vi "get Data Read.vi"(7 "data_pos":u16, 8 "error in (no error)":errorcluster, 9 "data_length":u16, 10 "protocol_version":i32, 11 "port_num":i32) -> (0 "error out":errorcluster, 3 "function return":u32)   [LabVIEW 2022 SP3, in "dxl.lvlib"]
doc: "WINDECLSPEC uint32_t getDataRead (int port_num, int protocol_version, uint16_t data_length, uint16_t data_pos);"
uses:
  dxl.lvlib
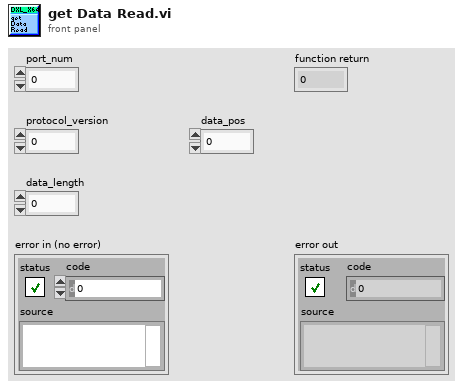
[diagram p1: front panel]
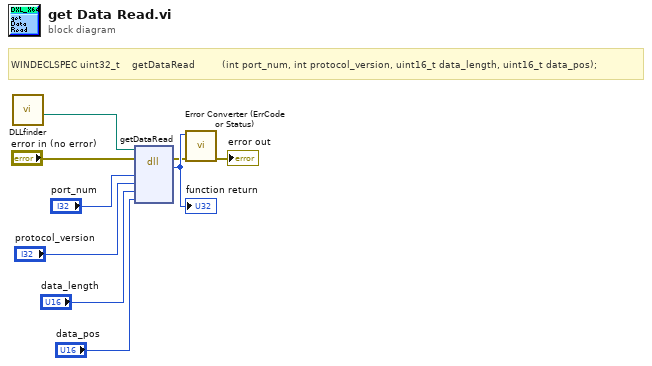
[diagram p0: block diagram]
diagram:
  # "WINDECLSPEC uint32_t    getDataRead         (int port_num, int protocol_version, uint16_t data_length, uint16_t data_pos);"
  n1 = call "DLLfinder.vi"() -> ("File Path"=w1:path)  [unwired: 11 in]
  n2 = dll-call lib="C:/EnFlo_Software/ADAM Serial/Instrument drivers/Dynamixel/2nd attempt/Library/dxl_x64_c.*" fn="getDataRead"(path in=w1, error in="error in (no error)", "port_num"="port_num", "protocol_version"="protocol_version", "data_length"="data_length", "data_pos"="data_pos") -> (error out=w3:errorcluster, "return type"=w9:u32)  [unwired: 5 in, 1 out]
  "function return" <- w9
  n3 = call "Error Converter (ErrCode or Status).vi"("error in (no error)"=w3, "error code"=w9) -> ("error out"=→"error out":errorcluster)  [unwired: 9 in]
